vi "sv_Frequency Range to Band Number.vi"(1 "frequency range [Hz]":cluster{"low freq.":dbl, "high freq.":dbl}={"low freq."=1000.0, "high freq."=1000.0} {"high freq." min=0.001 format="%.2f"; "low freq." min=0.001 format="%.2f"}, 2 "bandwidth":T2(ring)=enum."1/3 octave", 3 "standard":T1) -> (0 "band number":cluster{"low band":i32, "high band":i32})   [LabVIEW 2017, in "SoundVib_Octave_2014 standard.lvlib"]
doc: "Converts the selected frequency range to the corresponding band number, based on the specified bandwidth and standard (ANSI or IEC).\nThe band number is based on the low and high bands specified in the frequency range cluster. A value of 0 corresponds to the reference frequency of the audio-frequency range, 1 kHz. Each successive value corresponds to the next fractional-octave band. Positive values cover the range above 1 kHz, and negative values cover the range below 1 kHz."
uses:
  <vilib>/addons/Sound and Vibration/svt_Octave/SoundVib_Octave_2014 standard.lvlib
  <vilib>/addons/_NISVFA/_Shared subVIs/Controls/svc_Octave Standard.ctl
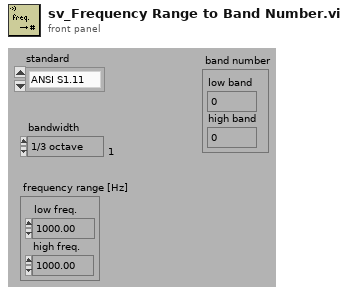
[diagram p1: front panel]
types:
  T1 = typedef "svc_Octave Standard.ctl" = enum16{"ANSI S1.11", "IEC 61260"}
  T2 = enum16{"1 octave", "1/3 octave", "1/6 octave", "1/12 octave", "1/24 octave", "1/48 octave", "1/96 octave"}
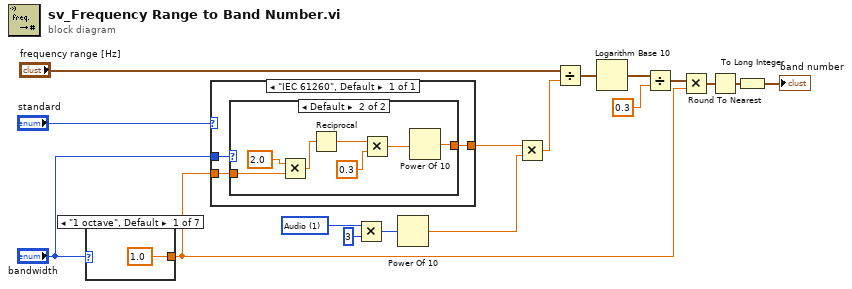
[diagram p0: block diagram]
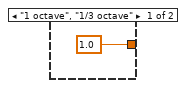
[diagram p2: hidden frame]
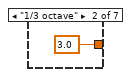
[diagram p3: hidden frame]
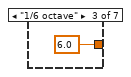
[diagram p4: hidden frame]
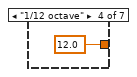
[diagram p5: hidden frame]
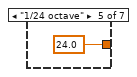
[diagram p6: hidden frame]
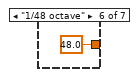
[diagram p7: hidden frame]
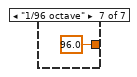
[diagram p8: hidden frame]
diagram:
  w13 = u16 1 items=["Infrasonic", "Audio", "Ultrasonic"] ("reference frequency range")
  n1 = case shown="\"1 octave\", Default" "bandwidth" {
    tunnel: [1.0 3.0 6.0 12.0 24.0 48.0 96.0] -> w9
    frame "1 octave", Default {
    }
    frame "1/3 octave" {
    }
    frame "1/6 octave" {
    }
    frame "1/12 octave" {
    }
    frame "1/24 octave" {
    }
    frame "1/48 octave" {
    }
    frame "1/96 octave" {
    }
  }
  n2 = case shown="\"IEC 61260\", Default" "standard" {
    tunnel: w9 -> [w27]
    tunnel: [w26] -> w8
    tunnel: "bandwidth" -> [w25]
    frame "IEC 61260", Default {
      n3 = case shown="Default" w25 {
        tunnel: [1.0 ("x") w35] -> w26
        tunnel: w27 -> [_ w33]
        frame "1 octave", "1/3 octave" {
        }
        frame Default {
          n4 = Multiply(x=2.0, y=w33) -> (x*y=w34:dbl)
          n5 = Reciprocal(x=w34) -> (1/x=w31:dbl)
          n6 = Multiply(x=w31, y=0.3 ("x")) -> (x*y=w29:dbl)
          n7 = Power Of 10(x=w29) -> (10^x=w35:dbl)
        }
      }
    }
  }
  n8 = Multiply(x=w13, y=u16 3) -> (x*y=w16:u16)
  n9 = Power Of 10(x=w16) -> (10^x=w14:dbl)
  n10 = Multiply(x=w8, y=w14) -> (x*y=w17:dbl)
  n11 = Divide(x="frequency range [Hz]", y=w17) -> (x/y=w7:cluster{"low freq.":dbl, "high freq.":dbl})
  n12 = Logarithm Base 10(1:w7) -> (0:w12:cluster{"low freq.":dbl, "high freq.":dbl})
  n13 = Divide(x=w12, y=0.3 ("x")) -> (x/y=w6:cluster{"low freq.":dbl, "high freq.":dbl})
  n14 = Multiply(x=w6, y=w9) -> (x*y=w11:cluster{"low freq.":dbl, "high freq.":dbl})
  n15 = Round To Nearest(number=w11) -> (nearest integer value=w10:cluster{"low freq.":dbl, "high freq.":dbl})
  n16 = To Long Integer(number=w10) -> (32bit integer=→"band number":cluster{"low freq.":i32, "high freq.":i32})
